vi "Graphics_Create.vi"(0 "reference":refnum<class "Graphics.lvclass">, 1 "screenRef":refnum<vi>, 5 "error in (no error)":errorcluster) -> (14 "reference out":refnum<class "Graphics.lvclass">, 19 "error out":errorcluster)   [LabVIEW 2014, in "Graphics.lvclass"]
doc: "Creates and initializes a new Graphics object.\n\nThis object should be destroyed using a Graphics destructor VI.\n\n[GOOP 2.4]"
uses:
  <resource>/Framework/Providers/Open_GDS/UML/Graphics_class/Graphics.lvclass
panel:
  # "The input reference should only\nbe wired when this method is called\nby a sub class constructor."
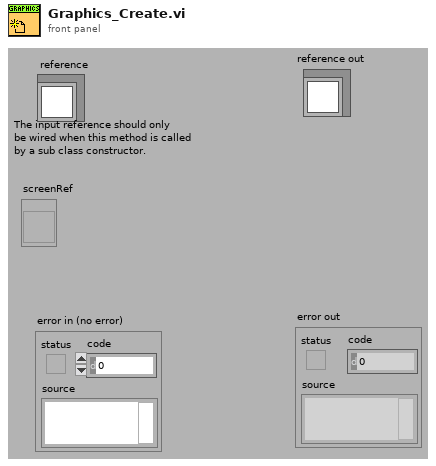
[diagram p1: front panel]
types:
  T1 = typedef "Graphics.lvclass/ObjectAttributes.ctl" = cluster{"drawColor":u32, "backgroundColor":u32, "font":T2, "fontType":T3, "picture":picture, "stroke":T4, "scaleX":dbl, "scaleY":dbl, "screenRef":refnum<vi>, "offsetX":dbl, "offsetY":dbl}
  T2 = typedef "Graphics.lvclass/FontType.ctl" = cluster{"Font Name:":string, "Size":i16, "Strikeout?":bool, "Italic?":bool, "Underline?":bool, "Outline?":bool, "Shadow?":bool, "Bold?":bool}
  T3 = typedef "Graphics.lvclass/LvFontType.ctl" = enum16{"User-specified Font", "Application Font", "System Font", "Dialog Font"}
  T4 = typedef "Graphics.lvclass/StrokeType.ctl" = enum16{"USE_DEFAULT", "SOLID", "DOTTED"}
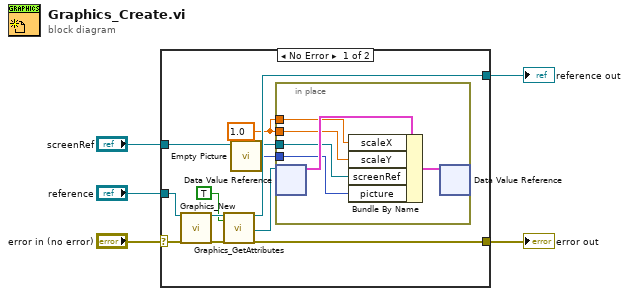
[diagram p0: block diagram]
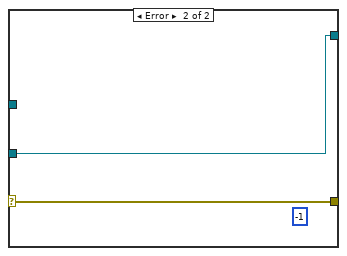
[diagram p2: hidden frame]
diagram:
  n1 = case shown="No Error" "error in (no error)" {
    selector: "error in (no error)" -> [w16 w24]
    tunnel: [w12 w23] -> w5
    tunnel: [w15 w24] -> w4
    tunnel: "reference" -> [w11 w23]
    tunnel: "screenRef" -> [w7 _]
    frame No Error {
      w8 = 1.0 ("scaleX")
      n2 = call <resource>:"Graphics_New.vi"("reference in"=w11, "error in (no error)"=w16) -> ("reference out"=w13:refnum<class "Graphics.lvclass">, "error out"=w14:errorcluster)  [unwired: 3 in, 13 out]
      n3 = call <resource>:"Graphics_GetAttributes.vi"("reference in"=w13, "OnlyGetDvrReference(False)"=TRUE, "error in (no error)"=w14) -> ("reference out"=w12:refnum<class "Graphics.lvclass">, "DataRef"=w9:refnum<data-value>, "error out"=w15:errorcluster)  [unwired: 13 in, 1 out]
      n4 = call "Empty Picture"() -> ("empty picture"=w6:picture)
      n5 = in-place {
        in-place-border: w8 -> [w21]
        in-place-border: w8 -> [w20]
        in-place-border: w7 -> [w19]
        in-place-border: w6 -> [w18]
        n6 = in-place-dvr #1(w9) -> (w22:T1)  [unwired: 1 out]
        n7 = Bundle By Name(cluster=w22, "scaleX"=w21, "scaleY"=w20, "screenRef"=w19, "picture"=w18) -> (w17:T1)
        n8 = in-place-dvr #1(w17) -> ()  [unwired: 2 out]
      }
    }
    frame Error {
      (unwired) -1 ("Nr of open handles")
    }
  }
  "error out" <- w4
  "reference out" <- w5
